vi "Configure Trigger Mode.vi"(8 "error in (no error)":errorcluster, 10 "Trigger Mode":T1=enum."Single Shot", 11 "Digital Delay Generator in":refnum<class "Digital Delay Generator.lvclass">) -> (0 "error out":errorcluster, 3 "Digital Delay Generator out":refnum<class "Digital Delay Generator.lvclass">)   [LabVIEW 2018, in "Digital Delay Generator.lvlib" / "Digital Delay Generator.lvclass"]
uses:
  Digital Delay Generator.lvclass
  Custom Controls/Trigger Mode.ctl
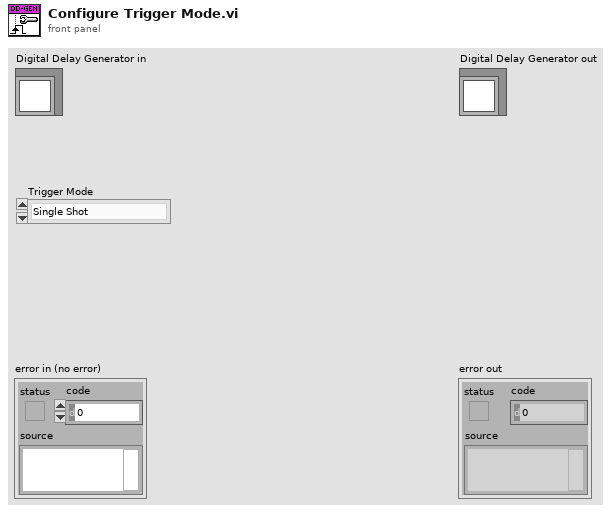
[diagram p1: front panel]
types:
  T1 = typedef "Digital Delay Generator.lvlib/Digital Delay Generator.lvclass/Trigger Mode.ctl" = enum16{"Internal", "External Rising Edge", "External Falling Edge", "Single Shot Internal Rising Edge", "Single Shot External Rising Edge", "Single Shot", "Line"}
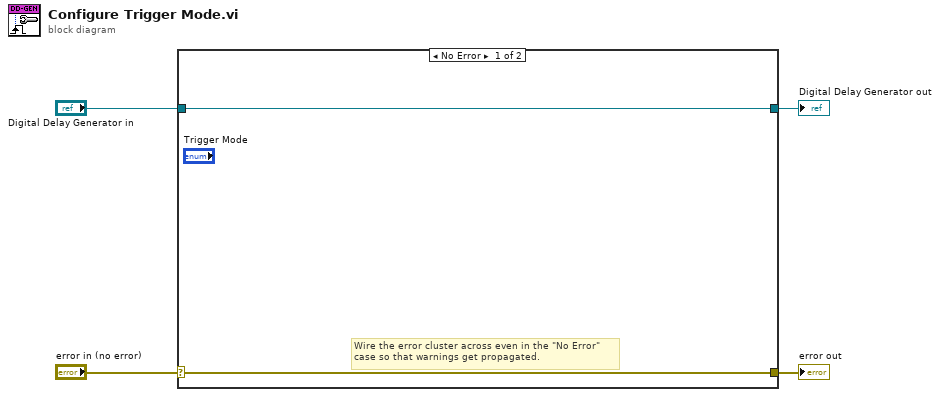
[diagram p0: block diagram]
diagram:
  n1 = case shown="No Error" "error in (no error)" {
    selector: "error in (no error)" -> [w5 w8]
    tunnel: [w5 w8] -> w3
    tunnel: [w6 w7] -> w1
    tunnel: "Digital Delay Generator in" -> [w6 w7]
    frame No Error {
      # "Wire the error cluster across even in the \"No Error\"\ncase so that warnings get propagated."
    }
    frame Error {
    }
  }
  "error out" <- w3
  "Digital Delay Generator out" <- w1
